vi "mb example client.vi"() -> ()   [LabVIEW 2013, in "Modbus Slave tests.lvlib"]
doc: "Platypus Framework 1.0.1.65\nNI Systems Engineering - National Instruments"
uses:
  Modbus Slave tests.lvlib
  <vilib>/NI/Modbus Library/API/Master/Modbus Master.lvclass
  <vilib>/NI/Modbus Library/API/Wrapper/Create TCP Master.vi
  <vilib>/NI/Modbus Library/API/Wrapper/API Main.lvlib
panel:
  out "D out":bool
  out "B out":dbl
  in  "C in":bool
  in  "A in":dbl
  in  "stop 2":bool
  out "final error":errorcluster
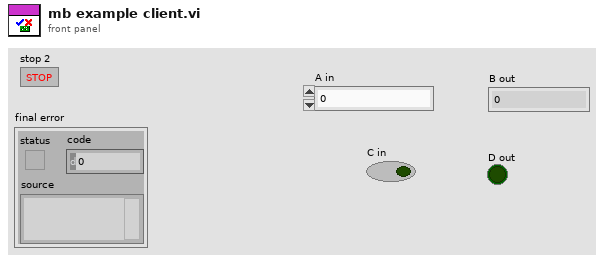
[diagram p1: front panel]
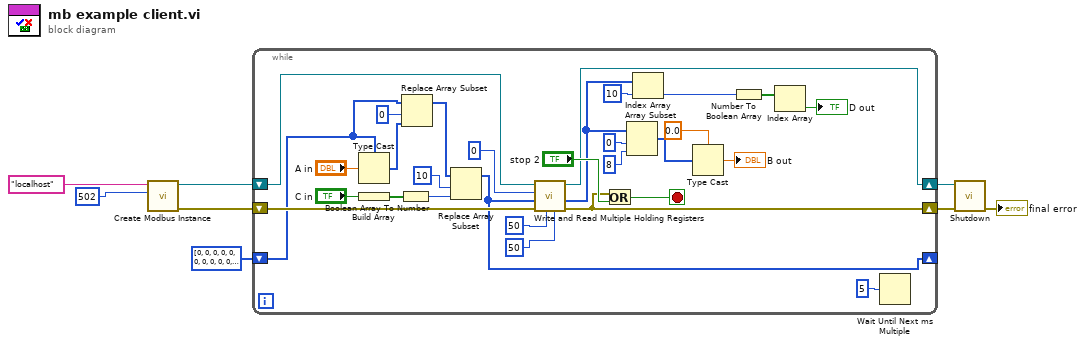
[diagram p0: block diagram]
diagram:
  n1 = call-poly <vilib>:"Create Modbus Instance.vi"("port (502)"=u16 502, "address"="localhost") -> ("error out"=w5:errorcluster, "TCP master instance"=w6:refnum<class "Modbus Master.lvclass">)  [unwired: 8 in]
  n2 = while {
    shift-right: [w33] -> w3
    shift-left: w6 -> [w35]
    shift-right: [w9] -> w4
    shift-left: w5 -> [w34]
    shift-right: [w29] -> _
    shift-left: u16[] [0, 0, 0, 0, 0, 0, 0, 0, 0, 0, 0, 0, 0, 0, 0, 0, 0, 0, 0, 0, 0, 0, 0, 0, 0, 0, 0, 0, 0, 0, 0, 0, 0, 0, 0, 0, 0, 0, 0, 0, 0, 0, 0, 0, 0, 0, 0, 0, 0, 0] ("write values") -> [w24]
    stop <- w36 stop-if-true
    n3 = Type Cast(type=w24, x="A in") -> (*(type *) &x=w23:u16[])
    n4 = Build Array("C in") -> (w21:bool[])
    n5 = Boolean Array To Number(Boolean array=w21) -> (number=w20:u16)
    n6 = Replace Array Subset(array=w24, new element=w23, index=0) -> (w28:u16[])
    n7 = Replace Array Subset(array=w28, new element=w20, index=10) -> (w29:u16[])
    n8 = call-dynamic "Write and Read Multiple Holding Registers.vi"("read count"=u16 50, "read starting address"=u16 50, "error in"=w34, "write values"=w29, "write starting address"=u16 0, "Modbus instance in"=w35) -> ("error out"=w9:errorcluster, "read values"=w14:u16[], "Modbus instance out"=w33:refnum<class "Modbus Master.lvclass">)  [unwired: 3 in]
    n9 = Or(x=w9, y="stop 2") -> (x .or. y?=w36:bool)
    n10 = Array Subset(array=w14, index=0, length=8) -> (w17:u16[])
    n11 = Index Array(array=w14, index=10) -> (element=w12:u16)
    n12 = Type Cast(type=0.0, x=w17) -> (*(type *) &x=→"B out":dbl)
    n13 = Number To Boolean Array(number=w12) -> (Boolean array=w11:bool[])
    n14 = Index Array(array=w11) -> (element=→"D out":bool)  [unwired: 1 in]
    n15 = Wait Until Next ms Multiple(millisecond multiple=u32 5) -> ()  [unwired: 1 out]
  }
  n16 = call-dynamic "Shutdown.vi"("error in"=w4, "Modbus master in"=w3) -> ("error out"=→"final error":errorcluster)  [unwired: 9 in]
